vi "pp_waitUntil.vi"(11 "until time":timestamp) -> ()   [LabVIEW 2013]
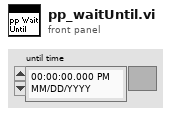
[diagram p1: front panel]
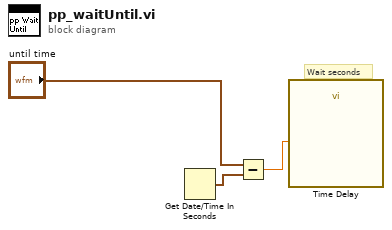
[diagram p0: block diagram]
diagram:
  # "Wait seconds"
  n1 = Get Date/Time In Seconds() -> (seconds since 1Jan1904=w2:timestamp)
  n2 = Subtract(x="until time", y=w2) -> (x-y=w3:dbl)
  n3 = call "Time Delay"("Delay Time (s)"=w3) -> ()  [unwired: 10 in, 1 out]
